vi "Read CSV.vi"(0 "file path (dialog if empty)":path) -> (1 "Time Data":dbl, 2 "ECG Data":dbl[](array[numeric]), 3 "Original ECG":waveform(dbl)(graph))   [LabVIEW 2018]
uses:
  <vilib>/Utility/file.llb/Read Delimited Spreadsheet (DBL).vi
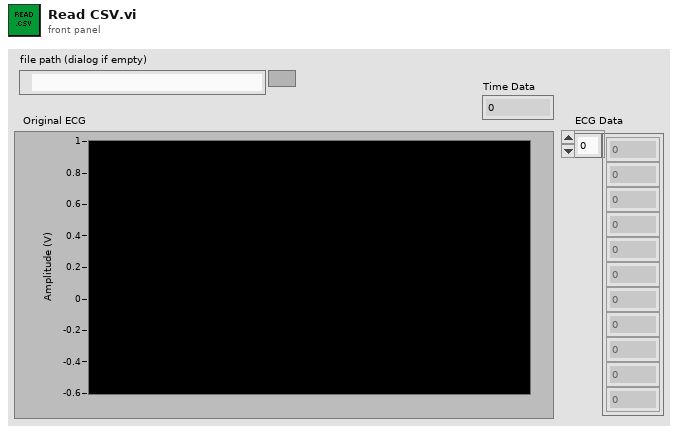
[diagram p1: front panel]
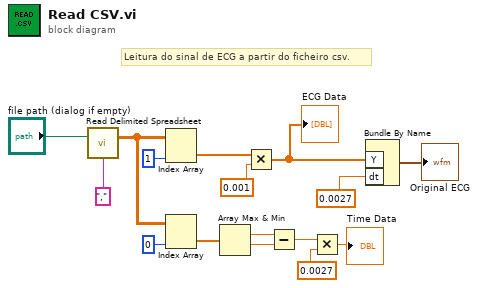
[diagram p0: block diagram]
diagram:
  # "Leitura do sinal de ECG a partir do ficheiro csv."
  n1 = call-poly <vilib>:"Read Delimited Spreadsheet.vi"("file path (dialog if empty)"="file path (dialog if empty)", "delimiter (\\t)"="," ("delimiter (\\t)")) -> ("all rows"=w13:dbl[][])  [unwired: 8 in, 5 out]
  n2 = Index Array(array=w13, index (col)=1 ("index (row)")) -> (element=w16:dbl[])  [unwired: 1 in]
  n3 = Index Array(array=w13, index (col)=0 ("disabled index (col)")) -> (element=w12:dbl[])  [unwired: 1 in]
  n4 = Array Max & Min(array=w12) -> (max value=w11:dbl, min value=w10:dbl)  [unwired: 2 out]
  n5 = Multiply(x=w16, y=0.001) -> (x*y=w14:dbl[])
  "ECG Data" <- w14
  n6 = Subtract(x=w11, y=w10) -> (x-y=w9:dbl)
  n7 = Multiply(x=w9, y=0.0027) -> (x*y=→"Time Data":dbl)
  n8 = Bundle By Name ("Build Waveform")("Y"=w14, "dt"=0.0027) -> (→"Original ECG":waveform(dbl))  [unwired: 1 in]
